vi "Execute Kernel Simple.vi"(8 "Error In":errorcluster, 9 "Kernel Handle":T2, 10 "Thread Dimensions":T1={"Depth"=1, "Height"=1, "Width"=1} {"Width" min=1; "Height" min=1; "Depth" min=1}, 11 "Device In":T3) -> (0 "Error Out":errorcluster, 1 "Kernel Handle out":T2, 3 "Device Out":T3, 4 "Time in ms":dbl)   [LabVIEW 2012]
doc: "Executes a kernel after all the arguments have been set. The width, height, and depth of each respective dimension depends on the type of kernel being executed. It is recommended to read the OpenCL standard to best know how to use these."
uses:
  Non-User VIs/Controls/Device ID.ctl
  Non-User VIs/Controls/Kernel Handle.ctl
  User Controls/Array Dimensions.ctl
  Non-User VIs/Error Checking/Add Error Functional Global.vi
  OpenCLV x64.lvlib
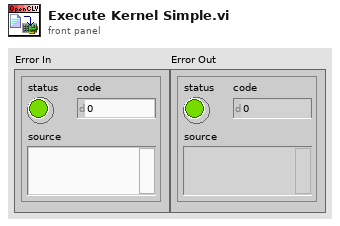
[diagram p1: front panel]
types:
  T1 = typedef "Array Dimensions.ctl" = cluster{"Depth":u64, "Height":u64, "Width":u64}
  T2 = typedef "OpenCLV x64.lvlib/Kernel Handle.ctl" = u64
  T3 = typedef "OpenCLV x64.lvlib/Device ID.ctl" = u64
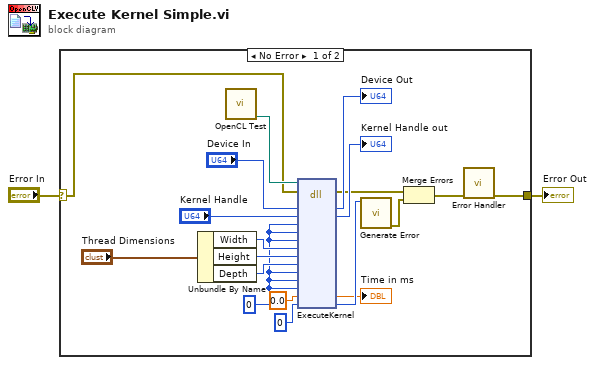
[diagram p0: block diagram]
diagram:
  n1 = case shown="No Error" "Error In" {
    selector: "Error In" -> [w3 w22]
    tunnel: [w4 w22] -> w1
    frame No Error {
      w10 = u64 0 ("Global Width Offset")
      n2 = Unbundle By Name("Thread Dimensions") -> ("Width"=w17:u64, "Height"=w16:u64, "Depth"=w15:u64)
      n3 = call "OpenCL Test.vi"() -> ("DLL To Use"=w6:path)  [unwired: 11 in]
      n4 = dll-call lib="C:/Users/bme-amcelroy-la/Desktop/OpenCLV/trunk/OpenCLV_x64_1.0/OpenCLV_x64.dll" fn="ExecuteKernel"(path in=w6, error in=w3, "Device In"="Device In", "Kernel"="Kernel Handle", "Global Width Offset"=w10, "Global Height Offset"=w10, "Global Depth Offset"=w10, "Global Width"=w17, "Global Height"=w16, "Global Depth"=w15, "Local Width"=w10, "Local Height"=w10, "Local Depth"=w10, "Time"=0.0, "Error"=0) -> (error out=w7:errorcluster, "Device In"=→"Device Out":u64, "Kernel"=→"Kernel Handle out":u64, "Time"=→"Time in ms":dbl, "Error"=w12:i32)  [unwired: 11 in, 1 out]
      n5 = call "Generate Error.vi"("Error"=w12) -> ("error out"=w8:errorcluster)  [unwired: 10 in]
      n6 = Merge Errors(w7, w8) -> (w5:errorcluster)
      n7 = call-poly "Error Handler.vi"("Error In"=w5) -> ("Error Out"=w4:errorcluster)  [unwired: 10 in]
    }
    frame Error {
    }
  }
  "Error Out" <- w1
